vi "task2.vi"() -> ()   [LabVIEW 2021]
uses:
  <vilib>/Utility/file.llb/Write Delimited Spreadsheet (DBL).vi
panel:
  out "Elapsed time":u32
  out "Sampling period (ms)":dbl
  out "Total number of samples":dbl
  in  "Sampling rate(Hz)":dbl
  in  "Total duration(s)":dbl
  out "sampled acquired":i32
  out "Waveform Graph":dbl[](graph)
  in  "file path (dialog if empty)":path
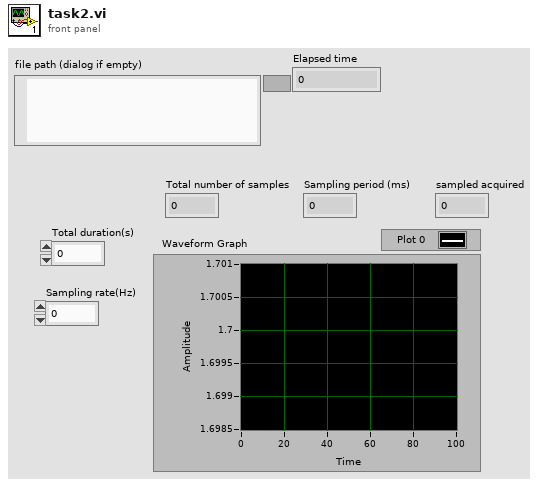
[diagram p1: front panel]
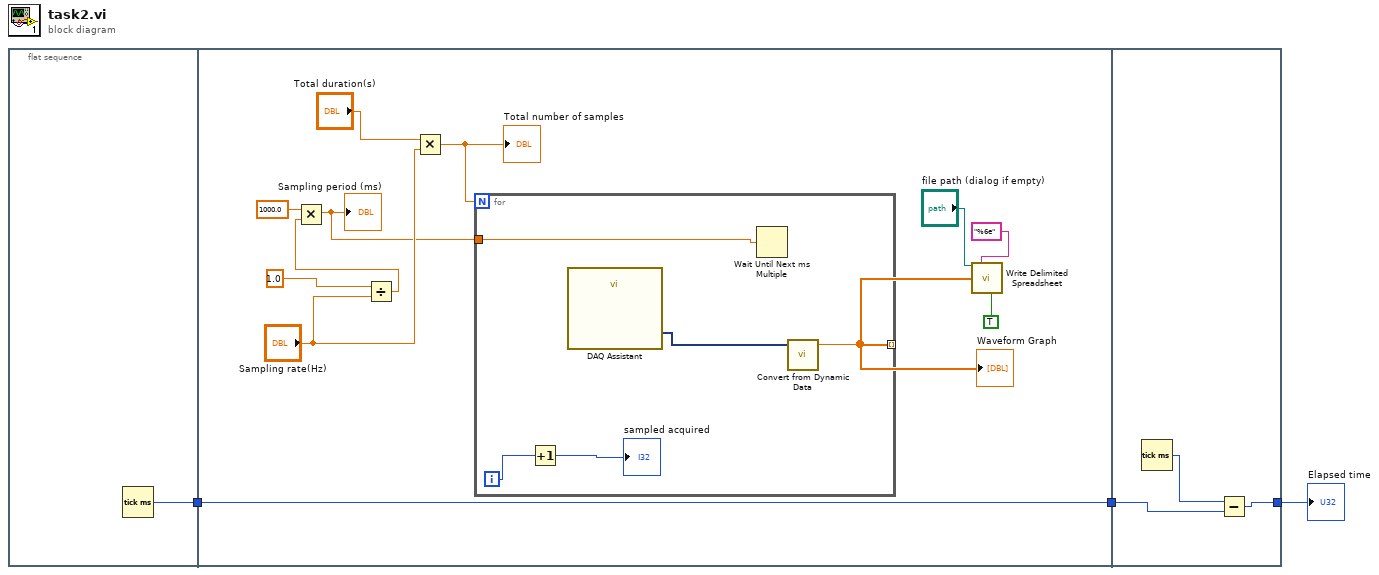
[diagram p0: block diagram]
diagram:
  n1 = flat-sequence {
    tunnel: [w4] -> w3
    tunnel: w3 -> [w5]
    tunnel: [w5] -> w2
    tunnel: w2 -> [w22]
    tunnel: [w24] -> w1
    frame #0 {
      n2 = Tick Count (ms)() -> (millisecond timer value=w4:u32)
    }
    frame #1 {
      n3 = Divide(x=1.0, y="Sampling rate(Hz)") -> (x/y=w8:dbl)
      n4 = Multiply(x=1000.0, y=w8) -> (x*y=w6:dbl)
      "Sampling period (ms)" <- w6
      n5 = Multiply(x="Total duration(s)", y="Sampling rate(Hz)") -> (x*y=w7:dbl)
      "Total number of samples" <- w7
      n6 = for {
        N: w7 -> [_]
        tunnel: [w21] -> w13 mode=indexing
        tunnel: w6 -> [w17]
        i -> [w20]
        n7 = Increment(x=w20) -> (x+1=→"sampled acquired":i32)
        n8 = call "DAQ Assistant"() -> ("data"=w18:dynamicdata)  [unwired: 17 in, 2 out]
        n9 = Wait Until Next ms Multiple(millisecond multiple=w17) -> ()  [unwired: 1 out]
        n10 = call "Convert from Dynamic Data"("Dynamic Data Type"=w18) -> ("Scalar"=w21:dbl)  [unwired: 3 in]
      }
      "Waveform Graph" <- w13
      n11 = call-poly <vilib>:"Write Delimited Spreadsheet.vi"("file path (dialog if empty)"="file path (dialog if empty)", "format (%.3f)"="%6e", "1D data"=w13, "transpose? (no:F)"=TRUE) -> ()  [unwired: 10 in, 2 out]
    }
    frame #2 {
      n12 = Tick Count (ms)() -> (millisecond timer value=w23:u32)
      n13 = Subtract(x=w23, y=w22) -> (x-y=w24:u32)
    }
  }
  "Elapsed time" <- w1
